vi "Get Wire Type.vi"(8 "error in (no error)":errorcluster, 11 "sfixed32 in":refnum<class "packed.lvclass">) -> (0 "error out":errorcluster, 2 "Wire Type":T1, 3 "sfixed32 out":refnum<class "packed.lvclass">)   [LabVIEW 2020, in "Protobuf RAW.lvlib" / "packed.lvclass"]
uses:
  packed.lvclass
  Type Serializer/Wire Type.ctl
  packed.lvclass/packed.ctl
  Wire Type Group/Wire Type Group.lvclass
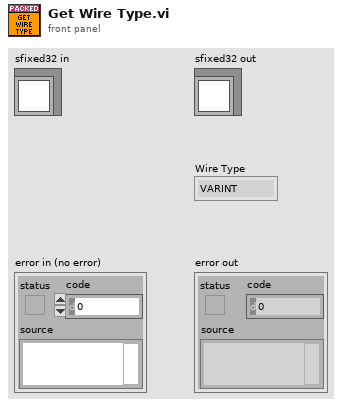
[diagram p1: front panel]
types:
  T1 = typedef "Protobuf RAW.lvlib/Wire Type Group.lvclass/Wire Type.ctl" = enum16{"VARINT", "I64", "LEN", "SGROUP", "EGROUP", "I32"}
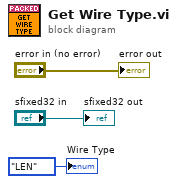
[diagram p0: block diagram]
diagram:
  "error out" <- "error in (no error)"
  "sfixed32 out" <- "sfixed32 in"
  "Wire Type" <- Wire_Type."LEN" ("Wire Type")
